vi "SetSyncTrigger.vi"(8 "error in (no error)":errorcluster, 9 "SyncLevel":i32=-100 caption="Level      mV" min=-1200 max=1200 step=1, 10 "SyncEdge":i32(ring) caption="Edge" items=["falling", "rising"], 11 "Multiharp in":refnum<class "Multiharp.lvclass">) -> (0 "error out":errorcluster, 3 "Multiharp out":refnum<class "Multiharp.lvclass">)   [LabVIEW 2023, in "Multiharp.lvlib" / "Multiharp.lvclass"]
uses:
  Multiharp.lvclass
  <vilib>/ActorFramework/Actor/Actor.lvclass
  Multiharp Messages/SetSyncOffset Msg/SetSyncOffset Msg.lvclass
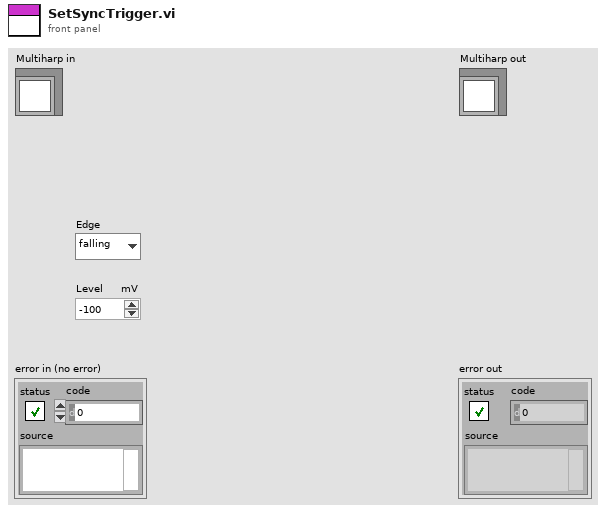
[diagram p1: front panel]
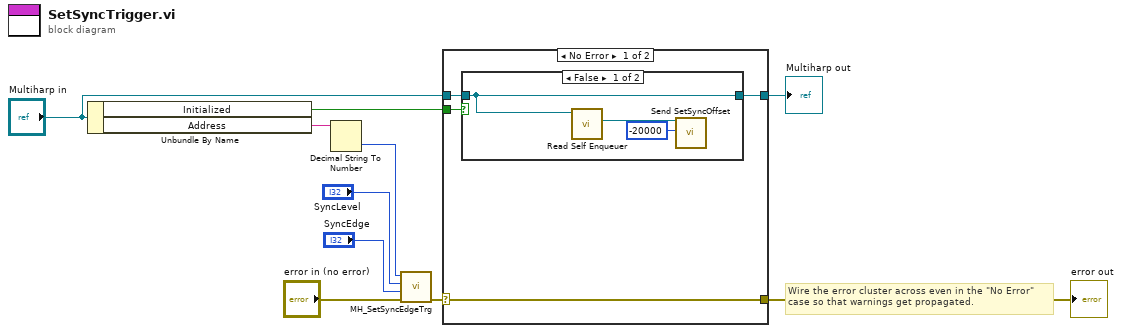
[diagram p0: block diagram]
diagram:
  # "Wire the error cluster across even in the \"No Error\"\ncase so that warnings get propagated."
  n1 = Unbundle By Name("Multiharp in") -> ("Initialized"=w5:bool, "Address"=w10:string)
  n2 = Decimal String To Number(string=w10) -> (number=w9:i32)  [unwired: 2 in, 1 out]
  n3 = call "MH_SetSyncEdgeTrg.vi"("error in (no error)"="error in (no error)", "edge"="SyncEdge", "level"="SyncLevel", "devidx"=w9) -> ("error out"=w6:errorcluster)  [unwired: 6 in, 1 out]
  n4 = case shown="No Error" w6 {
    selector: w6 -> [w11 w19]
    tunnel: w5 -> [w14 _]
    tunnel: "Multiharp in" -> [w13 w20]
    tunnel: [w12 w20] -> w3
    tunnel: [w11 w19] -> w1
    frame No Error {
      n5 = case shown="False" w14 {
        tunnel: w13 -> [w17 w18]
        tunnel: [w17 w18] -> w12
        frame False {
          n6 = call <vilib>:"Read Self Enqueuer.vi"("Actor"=w17) -> ("Self Enqueuer"=w16:refnum<class "Message Enqueuer.lvclass">)  [unwired: 10 in]
          n7 = call "Send SetSyncOffset.vi"("Offset"=-20000, "Message Enqueuer"=w16) -> ()  [unwired: 8 in, 2 out]
        }
        frame True {
          # "Send message to UI"
        }
      }
    }
    frame Error {
    }
  }
  "error out" <- w1
  "Multiharp out" <- w3
